vi "HP5313xA Initialize2023.vi"(1 "reset (T:yes)":bool, 2 "error in (no error)":errorcluster, 3 "GPIB Address":i16=10, 4 "GPIB Bus":i32) -> (0 "error out":errorcluster)   [LabVIEW 2023]
doc: "This VI loads the addressing information about the instrument into the Open Instrument VI and returns the instrument ID. You can reset the instrument by setting the front panel reset control. You must run this VI before using any of the instrument driver VIs for this instrument."
panel:
  # "yes\nno"
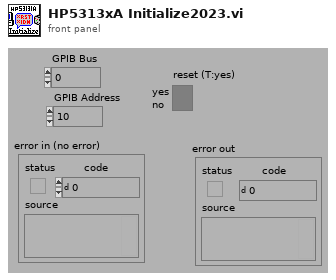
[diagram p1: front panel]
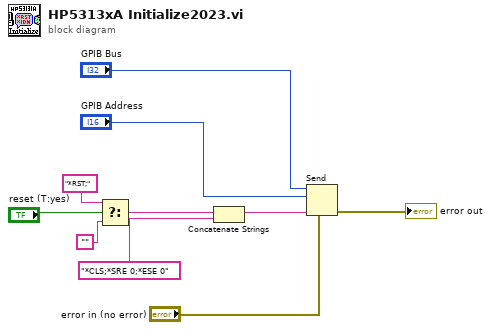
[diagram p0: block diagram]
diagram:
  n1 = Select(t="*RST;", s="reset (T:yes)", f="") -> (s? t:f=w7:string)
  n2 = Concatenate Strings(w7, "*CLS;*SRE 0;*ESE 0" ("data string")) -> (w5:string)
  n3 = Send(0:"GPIB Bus", 2:"GPIB Address", 4:"error in (no error)", 5:w5) -> (8:→"error out":errorcluster)  [unwired: 1 in, 2 out]
